vi "Autonomous Independent.vi"() -> ()   [LabVIEW 2014]
doc: "This VI is called when autonomous begins, and will automatically be terminated when autonomous ends. You can carry out timed or sensor driven robot movement independently without needing to return to the caller."
uses:
  <vilib>/Rock Robotics/WPI/Joystick/WPI_JoystickGetSetRefNum.vi
  <vilib>/Rock Robotics/WPI/RobotDrive/WPI_RobotDriveGetSetRefNum.vi
  <vilib>/Rock Robotics/WPI/RobotDrive/WPI_RobotDriveArcadeDrive_Standard(NoSaturation).vi
panel:
  out "Current Movement, for debugging":T1 {"Y Joystick Value" scale=1.0..-1.0; "X Joystick Value" scale=-1.0..1.0}
  in  "Array of robot movements":T2(array[cluster]) {"Y Joystick Value" scale=1.0..-1.0; "X Joystick Value" scale=-1.0..1.0}
  # "Be sure to right-click and choose Data Operations>>Make Current Value default if you want to save the array values with the VI"
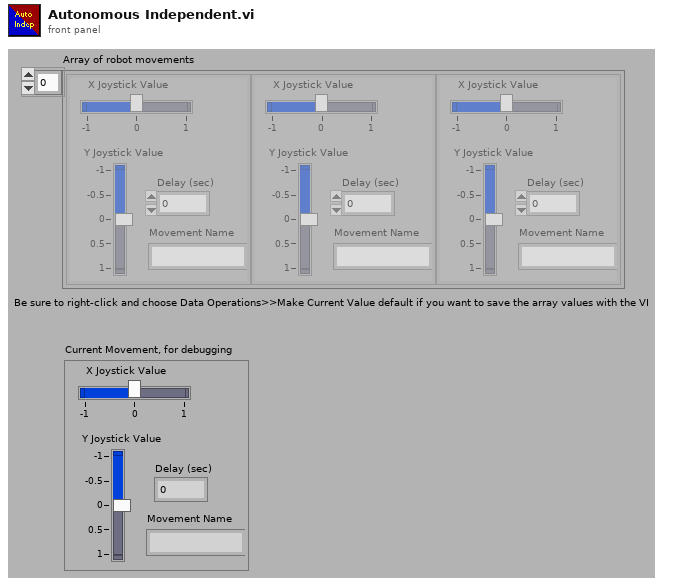
[diagram p1: front panel]
types:
  T1 = cluster{"X Joystick Value":dbl, "Y Joystick Value":dbl, "Delay (sec)":dbl, "Movement Name":string}
  T2 = cluster{"X Joystick Value":dbl, "Y Joystick Value":dbl, "Delay (sec)":dbl, "Movement Name":string}[]
  T3 = typedef "WPI_RobotDriveDevRef.ctl" = cluster{"DevStatus":errorcluster, "Motors[]":T4[], "Square Inputs":bool, "Max Output":dbl}
  T4 = typedef "WPI_MotorControlDeviceRef.ctl" = cluster{"DeviceStatus":errorcluster, "Type":T5, "PWM":cluster{"Controller":T6, "PWM Channel":T7, "DeadBand":T8}, "CAN":cluster{"Device Number":u8, "Control Mode":T9, "Semaphore":T10, "Max Vout":dbl, "TalonSRX Control Mode":T11}, "Invert":bool, "TransformRef":T12, "InvTransformRef":T12}
  T5 = typedef "WPI_MotorControlType.ctl" = enum16{"PWM", "CAN", "CANTalonSRX"}
  T6 = typedef "FPGA_TypedefDigitalModule.ctl" = enum16{"Controller 1"}
  T7 = typedef "FPGA_DIOPWMChannel.ctl" = enum8{"PWM 0", "PWM 1", "PWM 2", "PWM 3", "PWM 4", "PWM 5", "PWM 6", "PWM 7", "PWM 8", "PWM 9", "PWM MXP 0", "PWM MXP 1", "PWM MXP 2", "PWM MXP 3", "PWM MXP 4", "PWM MXP 5", "PWM MXP 6", "PWM MXP 7", "PWM MXP 8", "PWM MXP 9", "Invalid"}
  T8 = typedef "WPI_PWMDeadband.ctl" = cluster{"Name":string, "maxPositivePwm":i32, "minPositivePwm":i32, "centerPwm":i32, "maxNegativePwm":i32, "minNegativePwm":i32, "angularRange":u16}
  T9 = typedef "WPI_CANJaguar_ControlMode.ctl" = enum8{"Percent VBus", "Current", "Speed", "Position", "Voltage"}
  T10 = typedef "Semaphore RefNum" = refnum<k1>
  T11 = typedef "WPI_CANTalonSRX_APIControlMode.ctl" = enum8{"Percent VBus", "Speed", "Position", "Slave", "Unchanged / Invalid"}
  T12 = typedef "WPI_PWMTransform_ConPane.ctl" = refnum<vi>
  T13 = typedef "WPI_JoystickDevRef.ctl" = cluster{"Device":T14}
  T14 = typedef "WPI_JoystickDeviceEnum.ctl" = enum16{"USB 0", "USB 1", "USB 2", "USB 3", "USB 4", "USB 5"}
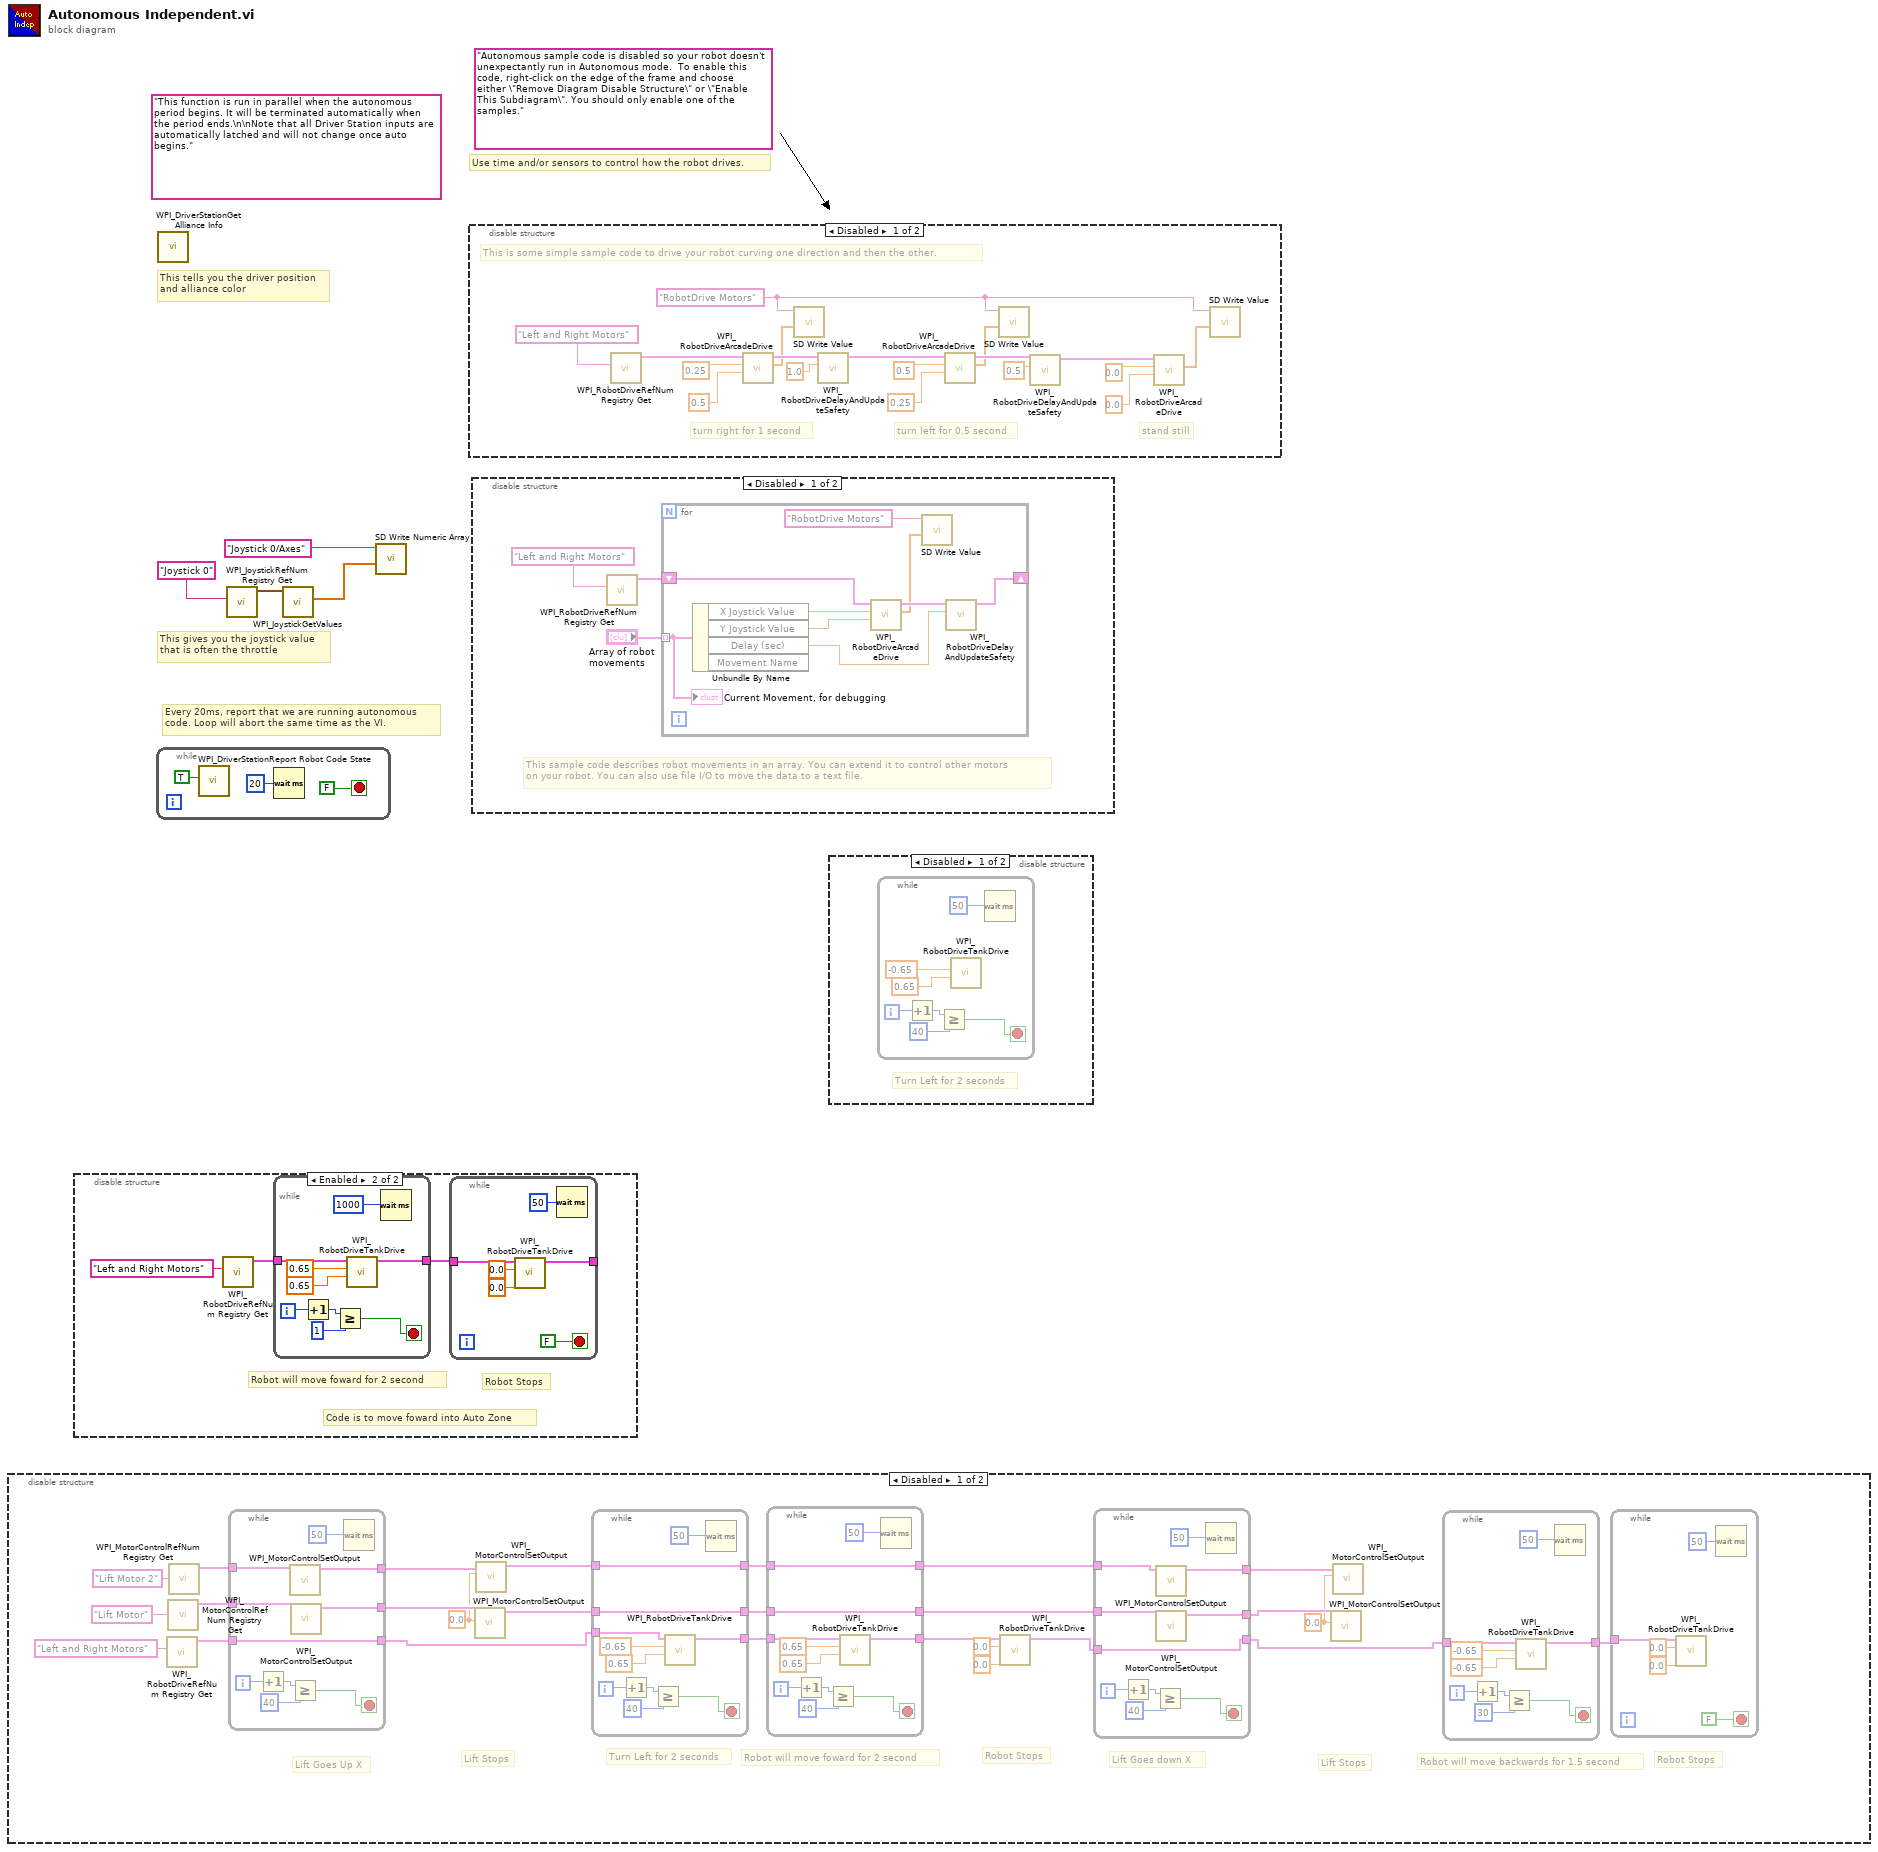
[diagram p0: block diagram]
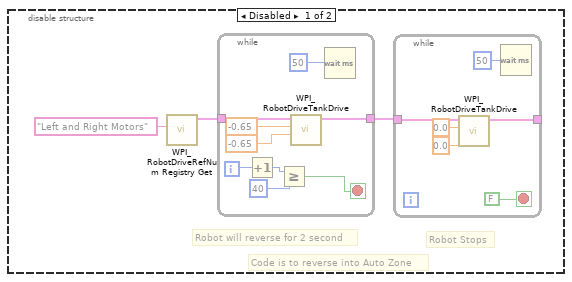
[diagram p4: hidden frame]
diagram:
  (unwired) "Autonomous sample code is disabled so your robot doesn't unexpectantly run in Autonomous mode.  To enable this code, right-click on the edge of the frame and choose either \"Remove Diagram Disable Structure\" or \"Enable This Subdiagram\". You should only enable one of the samples."
  (unwired) "This function is run in parallel when the autonomous period begins. It will be terminated automatically when the period ends.\n\nNote that all Driver Station inputs are automatically latched and will not change once auto begins."
  # "Every 20ms, report that we are running autonomous\ncode. Loop will abort the same time as the VI."
  # "This gives you the joystick value\nthat is often the throttle"
  # "Use time and/or sensors to control how the robot drives."
  # "This tells you the driver position\nand alliance color"
  n1 = disable-structure shown="Disabled" {
    frame Disabled {
      w5 = 0.0 ("Output")
      w8 = 0.0 ("Output")
      # "Lift Goes Up X"
      # "Lift Goes down X"
      # "Lift Stops"
      # "Lift Stops"
      # "Robot will move backwards for 1.5 second"
      # "Robot Stops"
      # "Turn Left for 2 seconds"
      # "Robot Stops"
      # "Robot will move foward for 2 second"
      n2 = call <vilib>:"WPI_RobotDriveRefNum Registry Get.vi"("refnum name"="Left and Right Motors") -> ("RobotDriveDevRef"=w25:T3)  [unwired: 9 in, 1 out]
      n3 = call <vilib>:"WPI_MotorControlRefNum Registry Get.vi"("refnum name"="Lift Motor") -> ("MotorControlDevRef"=w28:T4)  [unwired: 9 in, 1 out]
      n4 = call <vilib>:"WPI_MotorControlRefNum Registry Get.vi"("refnum name"="Lift Motor 2") -> ("MotorControlDevRef"=w14:T4)  [unwired: 9 in, 1 out]
      n5 = while {
        tunnel: w28 -> [w54]
        tunnel: [w53] -> w24
        tunnel: w25 -> [w52]
        tunnel: [w52] -> w22
        tunnel: w14 -> [w51]
        tunnel: [w50] -> w13
        i -> [w57]
        stop <- w56 stop-if-true
        n6 = Increment(x=w57) -> (x+1=w58:i32)
        n7 = call <vilib>:"WPI_MotorControlSetOutput.vi"("MotorControlDevRef"=w51) -> ("MotorControlDevRef"=w50:T4)  [unwired: 8 in, 2 out]
        n8 = Greater Or Equal?(x=w58, y=40) -> (x >= y?=w56:bool)
        n9 = call <vilib>:"WPI_MotorControlSetOutput.vi"("MotorControlDevRef"=w54) -> ("MotorControlDevRef"=w53:T4)  [unwired: 8 in, 2 out]
        n10 = Wait (ms)(milliseconds to wait=u32 50) -> ()  [unwired: 1 out]
      }
      n11 = call <vilib>:"WPI_MotorControlSetOutput.vi"("Output"=w5, "MotorControlDevRef"=w24) -> ("MotorControlDevRef"=w23:T4)  [unwired: 7 in, 2 out]
      n12 = call <vilib>:"WPI_MotorControlSetOutput.vi"("Output"=w5, "MotorControlDevRef"=w13) -> ("MotorControlDevRef"=w10:T4)  [unwired: 7 in, 2 out]
      n13 = while {
        tunnel: [w63] -> w29
        tunnel: w23 -> [w62]
        tunnel: [w62] -> w27
        tunnel: w22 -> [w61]
        tunnel: [w60] -> w11
        tunnel: w10 -> [w60]
        i -> [w68]
        stop <- w67 stop-if-true
        n14 = Increment(x=w68) -> (x+1=w69:i32)
        n15 = Greater Or Equal?(x=w69, y=40) -> (x >= y?=w67:bool)
        n16 = call <vilib>:"WPI_RobotDriveTankDrive.vi"("Right axis value"=0.65, "Left axis value"=-0.65, "RobotDriveDevRef"=w61) -> ("RobotDriveDevRef"=w63:T3)  [unwired: 6 in, 2 out]
        n17 = Wait (ms)(milliseconds to wait=u32 50) -> ()  [unwired: 1 out]
      }
      n18 = while {
        tunnel: w29 -> [w81]
        tunnel: [w78] -> w21
        tunnel: w27 -> [w77]
        tunnel: [w77] -> w19
        tunnel: [w76] -> w12
        tunnel: w11 -> [w76]
        i -> [w84]
        stop <- w83 stop-if-true
        n19 = Increment(x=w84) -> (x+1=w85:i32)
        n20 = Greater Or Equal?(x=w85, y=40) -> (x >= y?=w83:bool)
        n21 = call <vilib>:"WPI_RobotDriveTankDrive.vi"("Right axis value"=0.65, "Left axis value"=0.65, "RobotDriveDevRef"=w81) -> ("RobotDriveDevRef"=w78:T3)  [unwired: 6 in, 2 out]
        n22 = Wait (ms)(milliseconds to wait=u32 50) -> ()  [unwired: 1 out]
      }
      n23 = call <vilib>:"WPI_RobotDriveTankDrive.vi"("Right axis value"=0.0, "Left axis value"=0.0, "RobotDriveDevRef"=w21) -> ("RobotDriveDevRef"=w20:T3)  [unwired: 6 in, 2 out]
      n24 = while {
        tunnel: w19 -> [w44]
        tunnel: [w43] -> w17
        tunnel: w20 -> [w43]
        tunnel: [w42] -> w18
        tunnel: w12 -> [w41]
        tunnel: [w40] -> w9
        i -> [w47]
        stop <- w46 stop-if-true
        n25 = Increment(x=w47) -> (x+1=w48:i32)
        n26 = Greater Or Equal?(x=w48, y=40) -> (x >= y?=w46:bool)
        n27 = call <vilib>:"WPI_MotorControlSetOutput.vi"("MotorControlDevRef"=w41) -> ("MotorControlDevRef"=w40:T4)  [unwired: 8 in, 2 out]
        n28 = call <vilib>:"WPI_MotorControlSetOutput.vi"("MotorControlDevRef"=w44) -> ("MotorControlDevRef"=w42:T4)  [unwired: 8 in, 2 out]
        n29 = Wait (ms)(milliseconds to wait=u32 50) -> ()  [unwired: 1 out]
      }
      n30 = call <vilib>:"WPI_MotorControlSetOutput.vi"("Output"=w8, "MotorControlDevRef"=w18) -> ()  [unwired: 7 in, 3 out]
      n31 = call <vilib>:"WPI_MotorControlSetOutput.vi"("Output"=w8, "MotorControlDevRef"=w9) -> ()  [unwired: 7 in, 3 out]
      n32 = while {
        tunnel: w17 -> [w34]
        tunnel: [w31] -> w16
        i -> [w37]
        stop <- w36 stop-if-true
        n33 = Increment(x=w37) -> (x+1=w38:i32)
        n34 = Greater Or Equal?(x=w38, y=30) -> (x >= y?=w36:bool)
        n35 = call <vilib>:"WPI_RobotDriveTankDrive.vi"("Right axis value"=-0.65, "Left axis value"=-0.65, "RobotDriveDevRef"=w34) -> ("RobotDriveDevRef"=w31:T3)  [unwired: 6 in, 2 out]
        n36 = Wait (ms)(milliseconds to wait=u32 50) -> ()  [unwired: 1 out]
      }
      n37 = while {
        tunnel: w16 -> [w74]
        stop <- FALSE stop-if-true
        n38 = call <vilib>:"WPI_RobotDriveTankDrive.vi"("Right axis value"=0.0, "Left axis value"=0.0, "RobotDriveDevRef"=w74) -> ()  [unwired: 6 in, 3 out]
        n39 = Wait (ms)(milliseconds to wait=u32 50) -> ()  [unwired: 1 out]
      }
    }
    frame Enabled {
    }
  }
  n40 = disable-structure shown="Enabled" {
    frame Disabled {
      # "Code is to reverse into Auto Zone"
      # "Robot Stops"
      # "Robot will reverse for 2 second"
      n41 = call <vilib>:"WPI_RobotDriveRefNum Registry Get.vi"("refnum name"="Left and Right Motors") -> ("RobotDriveDevRef"=w89:T3)  [unwired: 9 in, 1 out]
      n42 = while {
        tunnel: w89 -> [w99]
        tunnel: [w96] -> w87
        i -> [w102]
        stop <- w101 stop-if-true
        n43 = Increment(x=w102) -> (x+1=w103:i32)
        n44 = Greater Or Equal?(x=w103, y=40) -> (x >= y?=w101:bool)
        n45 = call <vilib>:"WPI_RobotDriveTankDrive.vi"("Right axis value"=-0.65, "Left axis value"=-0.65, "RobotDriveDevRef"=w99) -> ("RobotDriveDevRef"=w96:T3)  [unwired: 6 in, 2 out]
        n46 = Wait (ms)(milliseconds to wait=u32 50) -> ()  [unwired: 1 out]
      }
      n47 = while {
        tunnel: w87 -> [w94]
        tunnel: [w93] -> _
        stop <- FALSE stop-if-true
        n48 = call <vilib>:"WPI_RobotDriveTankDrive.vi"("Right axis value"=0.0, "Left axis value"=0.0, "RobotDriveDevRef"=w94) -> ("RobotDriveDevRef"=w93:T3)  [unwired: 6 in, 2 out]
        n49 = Wait (ms)(milliseconds to wait=u32 50) -> ()  [unwired: 1 out]
      }
    }
    frame Enabled {
      # "Robot Stops"
      # "Robot will move foward for 2 second"
      # "Code is to move foward into Auto Zone"
      n50 = call <vilib>:"WPI_RobotDriveRefNum Registry Get.vi"("refnum name"="Left and Right Motors") -> ("RobotDriveDevRef"=w105:T3)  [unwired: 9 in, 1 out]
      n51 = while {
        tunnel: w105 -> [w117]
        tunnel: [w114] -> w107
        i -> [w120]
        stop <- w119 stop-if-true
        n52 = Increment(x=w120) -> (x+1=w121:i32)
        n53 = Greater Or Equal?(x=w121, y=1) -> (x >= y?=w119:bool)
        n54 = call <vilib>:"WPI_RobotDriveTankDrive.vi"("Right axis value"=0.65, "Left axis value"=0.65, "RobotDriveDevRef"=w117) -> ("RobotDriveDevRef"=w114:T3)  [unwired: 6 in, 2 out]
        n55 = Wait (ms)(milliseconds to wait=u32 1000) -> ()  [unwired: 1 out]
      }
      n56 = while {
        tunnel: w107 -> [w112]
        tunnel: [w111] -> _
        stop <- FALSE stop-if-true
        n57 = call <vilib>:"WPI_RobotDriveTankDrive.vi"("Right axis value"=0.0, "Left axis value"=0.0, "RobotDriveDevRef"=w112) -> ("RobotDriveDevRef"=w111:T3)  [unwired: 6 in, 2 out]
        n58 = Wait (ms)(milliseconds to wait=u32 50) -> ()  [unwired: 1 out]
      }
    }
  }
  n59 = while {
    stop <- FALSE stop-if-true
    n60 = call <vilib>:"WPI_DriverStationReport Robot Code State.vi"("Autonomous"=TRUE) -> ()  [unwired: 10 in, 1 out]
    n61 = Wait (ms)(milliseconds to wait=u32 20) -> ()  [unwired: 1 out]
  }
  n62 = call <vilib>:"WPI_DriverStationGet Alliance Info.vi"() -> ()  [unwired: 12 out]
  n63 = call <vilib>:"WPI_JoystickRefNum Registry Get.vi"("refnum name"="Joystick 0") -> ("JoystickDevRef"=w3:T13)  [unwired: 1 in, 9 out]
  n64 = call <vilib>:"WPI_JoystickGetValues.vi"("JoystickDevRef"=w3) -> ("Axes"=w1:dbl[])  [unwired: 6 in, 4 out]
  n65 = call <vilib>:"SD Write Numeric Array.vi"("Numeric Array"=w1, "Name"="Joystick 0/Axes") -> ()  [unwired: 8 in, 2 out]
  n66 = disable-structure shown="Disabled" {
    frame Disabled {
      w129 = "RobotDrive Motors" ("Name")
      # "This is some simple sample code to drive your robot curving one direction and then the other."
      # "stand still"
      # "turn left for 0.5 second"
      # "turn right for 1 second"
      n67 = call <vilib>:"WPI_RobotDriveRefNum Registry Get.vi"("refnum name"="Left and Right Motors") -> ("RobotDriveDevRef"=w130:T3)  [unwired: 1 in, 9 out]
      n68 = call-poly <vilib>:"WPI_RobotDriveArcadeDrive.vi"("Y axis value"=0.5 ("X axis value"), "X axis value"=0.25, "RobotDriveDevRef"=w130) -> ("Motor Values"=w128:dbl[], "RobotDriveDevRef"=w137:T3)  [unwired: 1 in, 6 out]
      n69 = call-poly <vilib>:"SD Write Value.vi"("Numeric Array"=w128, "Name"=w129) -> ()  [unwired: 8 in, 2 out]
      n70 = call <vilib>:"WPI_RobotDriveDelayAndUpdateSafety.vi"("Delay (s)"=1.0, "RobotDriveDevRef"=w137) -> ("RobotDriveDevRef 2"=w136:T3)  [unwired: 8 in, 1 out]
      n71 = call-poly <vilib>:"WPI_RobotDriveArcadeDrive.vi"("Y axis value"=0.25 ("X axis value"), "X axis value"=0.5, "RobotDriveDevRef"=w136) -> ("Motor Values"=w127:dbl[], "RobotDriveDevRef"=w135:T3)  [unwired: 1 in, 6 out]
      n72 = call-poly <vilib>:"SD Write Value.vi"("Numeric Array"=w127, "Name"=w129) -> ()  [unwired: 8 in, 2 out]
      n73 = call <vilib>:"WPI_RobotDriveDelayAndUpdateSafety.vi"("Delay (s)"=0.5, "RobotDriveDevRef"=w135) -> ("RobotDriveDevRef 2"=w134:T3)  [unwired: 8 in, 1 out]
      n74 = call-poly <vilib>:"WPI_RobotDriveArcadeDrive.vi"("Y axis value"=0.0 ("X axis value"), "X axis value"=0.0, "RobotDriveDevRef"=w134) -> ("Motor Values"=w126:dbl[])  [unwired: 1 in, 7 out]
      n75 = call-poly <vilib>:"SD Write Value.vi"("Numeric Array"=w126, "Name"=w129) -> ()  [unwired: 8 in, 2 out]
    }
    frame Enabled {
    }
  }
  n76 = disable-structure shown="Disabled" {
    frame Disabled {
      # "This sample code describes robot movements in an array. You can extend it to control other motors\non your robot. You can also use file I/O to move the data to a text file."
      n77 = call <vilib>:"WPI_RobotDriveRefNum Registry Get.vi"("refnum name"="Left and Right Motors") -> ("RobotDriveDevRef"=w145:T3)  [unwired: 1 in, 9 out]
      n78 = for {
        shift-right: [w152] -> _
        shift-left: w145 -> [w153]
        tunnel: "Array of robot movements" -> [w148] mode=indexing
        n79 = Unbundle By Name(w148) -> ("X Joystick Value"=w151:dbl, "Y Joystick Value"=w150:dbl, "Delay (sec)"=w149:dbl)  [unwired: 1 out]
        n80 = call-poly <vilib>:"WPI_RobotDriveArcadeDrive.vi"("Y axis value"=w150, "X axis value"=w151, "RobotDriveDevRef"=w153) -> ("Motor Values"=w147:dbl[], "RobotDriveDevRef"=w154:T3)  [unwired: 1 in, 6 out]
        n81 = call-poly <vilib>:"SD Write Value.vi"("Numeric Array"=w147, "Name"="RobotDrive Motors") -> ()  [unwired: 8 in, 2 out]
        n82 = call <vilib>:"WPI_RobotDriveDelayAndUpdateSafety.vi"("Delay (s)"=w149, "RobotDriveDevRef"=w154) -> ("RobotDriveDevRef 2"=w152:T3)  [unwired: 8 in, 1 out]
        "Current Movement, for debugging" <- w148
      }
    }
    frame Enabled {
    }
  }
  n83 = disable-structure shown="Disabled" {
    frame Disabled {
      # "Turn Left for 2 seconds"
      n84 = while {
        i -> [w160]
        stop <- w159 stop-if-true
        n85 = Increment(x=w160) -> (x+1=w161:i32)
        n86 = Greater Or Equal?(x=w161, y=40) -> (x >= y?=w159:bool)
        n87 = call <vilib>:"WPI_RobotDriveTankDrive.vi"("Right axis value"=0.65, "Left axis value"=-0.65) -> ()  [unwired: 7 in, 3 out]
        n88 = Wait (ms)(milliseconds to wait=u32 50) -> ()  [unwired: 1 out]
      }
    }
    frame Enabled {
    }
  }
